vi "VI Tree.vi"   [LabVIEW 2025, in "Chroma 19052.lvlib"]
doc: "This is the instrument driver for the <INSTRUMENT NAME>. The VI Tree displays all the user-callable VIs of the instrument driver in an organized table."
uses:
  <instrlib>/Chroma 19052/Chroma 19052.lvlib
panel:
  # "(c) 2014 <Enter Company Name Here>.  ALL RIGHTS RESERVED."
  # "SEE DIAGRAM\nFOR VI TREE."
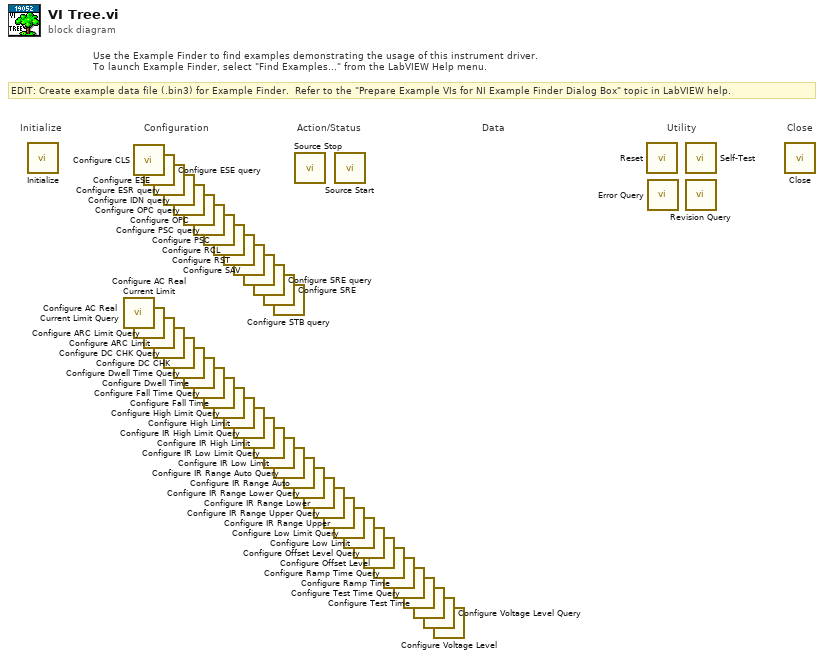
[diagram p0: block diagram]
diagram:
  # "EDIT: Create example data file (.bin3) for Example Finder.  Refer to the \"Prepare Example VIs for NI Example Finder Dialog Box\" topic in LabVIEW help."
  # "Use the Example Finder to find examples demonstrating the usage of this instrument driver.\nTo launch Example Finder, select \"Find Examples...\" from the LabVIEW Help menu."
  # "Configuration"
  # "Utility"
  # "Data"
  # "Action/Status"
  # "Close"
  # "Initialize"
  n1 = call <instrlib>:"Initialize.vi"() -> ()  [unwired: 10 in, 2 out]
  n2 = call <instrlib>:"Configure AC Real Current Limit Query.vi"() -> ()  [unwired: 8 in, 3 out]
  n3 = call <instrlib>:"Configure CLS.vi"() -> ()  [unwired: 10 in, 2 out]
  n4 = call <instrlib>:"Configure AC Real Current Limit.vi"() -> ()  [unwired: 9 in, 2 out]
  n5 = call <instrlib>:"Configure ESE query.vi"() -> ()  [unwired: 9 in, 3 out]
  n6 = call <instrlib>:"Configure ARC Limit Query.vi"() -> ()  [unwired: 9 in, 3 out]
  n7 = call <instrlib>:"Configure ESE.vi"() -> ()  [unwired: 10 in, 2 out]
  n8 = call <instrlib>:"Configure ARC Limit.vi"() -> ()  [unwired: 10 in, 2 out]
  n9 = call <instrlib>:"Configure ESR query.vi"() -> ()  [unwired: 9 in, 3 out]
  n10 = call <instrlib>:"Configure DC CHK Query.vi"() -> ()  [unwired: 10 in, 2 out]
  n11 = call <instrlib>:"Configure IDN query.vi"() -> ()  [unwired: 9 in, 3 out]
  n12 = call <instrlib>:"Configure DC CHK.vi"() -> ()  [unwired: 10 in, 2 out]
  n13 = call <instrlib>:"Configure OPC query.vi"() -> ()  [unwired: 9 in, 3 out]
  n14 = call <instrlib>:"Configure Dwell Time Query.vi"() -> ()  [unwired: 9 in, 3 out]
  n15 = call <instrlib>:"Configure OPC.vi"() -> ()  [unwired: 10 in, 2 out]
  n16 = call <instrlib>:"Configure Dwell Time.vi"() -> ()  [unwired: 10 in, 2 out]
  n17 = call <instrlib>:"Configure PSC query.vi"() -> ()  [unwired: 9 in, 3 out]
  n18 = call <instrlib>:"Configure Fall Time Query.vi"() -> ()  [unwired: 9 in, 3 out]
  n19 = call <instrlib>:"Configure PSC.vi"() -> ()  [unwired: 10 in, 2 out]
  n20 = call <instrlib>:"Configure Fall Time.vi"() -> ()  [unwired: 10 in, 2 out]
  n21 = call <instrlib>:"Configure RCL.vi"() -> ()  [unwired: 10 in, 2 out]
  n22 = call <instrlib>:"Configure High Limit Query.vi"() -> ()  [unwired: 9 in, 3 out]
  n23 = call <instrlib>:"Configure RST.vi"() -> ()  [unwired: 10 in, 2 out]
  n24 = call <instrlib>:"Configure High Limit.vi"() -> ()  [unwired: 10 in, 2 out]
  n25 = call <instrlib>:"Configure SAV.vi"() -> ()  [unwired: 10 in, 2 out]
  n26 = call <instrlib>:"Configure IR High Limit Query.vi"() -> ()  [unwired: 9 in, 3 out]
  n27 = call <instrlib>:"Configure SRE query.vi"() -> ()  [unwired: 9 in, 3 out]
  n28 = call <instrlib>:"Configure IR High Limit.vi"() -> ()  [unwired: 10 in, 2 out]
  n29 = call <instrlib>:"Configure SRE.vi"() -> ()  [unwired: 10 in, 2 out]
  n30 = call <instrlib>:"Configure IR Low Limit Query.vi"() -> ()  [unwired: 9 in, 3 out]
  n31 = call <instrlib>:"Configure STB query.vi"() -> ()  [unwired: 9 in, 3 out]
  n32 = call <instrlib>:"Configure IR Low Limit.vi"() -> ()  [unwired: 10 in, 2 out]
  n33 = call <instrlib>:"Configure IR Range Auto Query.vi"() -> ()  [unwired: 9 in, 3 out]
  n34 = call <instrlib>:"Configure IR Range Auto.vi"() -> ()  [unwired: 10 in, 2 out]
  n35 = call <instrlib>:"Source Stop.vi"() -> ()  [unwired: 10 in, 2 out]
  n36 = call <instrlib>:"Configure IR Range Lower Query.vi"() -> ()  [unwired: 9 in, 3 out]
  n37 = call <instrlib>:"Configure IR Range Lower.vi"() -> ()  [unwired: 10 in, 2 out]
  n38 = call <instrlib>:"Configure IR Range Upper Query.vi"() -> ()  [unwired: 9 in, 3 out]
  n39 = call <instrlib>:"Configure IR Range Upper.vi"() -> ()  [unwired: 10 in, 2 out]
  n40 = call <instrlib>:"Source Start.vi"() -> ()  [unwired: 10 in, 2 out]
  n41 = call <instrlib>:"Configure Low Limit Query.vi"() -> ()  [unwired: 9 in, 3 out]
  n42 = call <instrlib>:"Configure Low Limit.vi"() -> ()  [unwired: 10 in, 2 out]
  n43 = call <instrlib>:"Configure Offset Level Query.vi"() -> ()  [unwired: 10 in, 2 out]
  n44 = call <instrlib>:"Configure Offset Level.vi"() -> ()  [unwired: 10 in, 2 out]
  n45 = call <instrlib>:"Configure Ramp Time Query.vi"() -> ()  [unwired: 9 in, 3 out]
  n46 = call <instrlib>:"Configure Ramp Time.vi"() -> ()  [unwired: 10 in, 2 out]
  n47 = call <instrlib>:"Configure Test Time Query.vi"() -> ()  [unwired: 9 in, 3 out]
  n48 = call <instrlib>:"Configure Test Time.vi"() -> ()  [unwired: 10 in, 2 out]
  n49 = call <instrlib>:"Configure Voltage Level Query.vi"() -> ()  [unwired: 9 in, 3 out]
  n50 = call <instrlib>:"Configure Voltage Level.vi"() -> ()  [unwired: 10 in, 2 out]
  n51 = call <instrlib>:"Reset.vi"() -> ()  [unwired: 10 in, 2 out]
  n52 = call <instrlib>:"Error Query.vi"() -> ()  [unwired: 8 in, 4 out]
  n53 = call <instrlib>:"Self-Test.vi"() -> ()  [unwired: 8 in, 4 out]
  n54 = call <instrlib>:"Revision Query.vi"() -> ()  [unwired: 8 in, 4 out]
  n55 = call <instrlib>:"Close.vi"() -> ()  [unwired: 11 in, 1 out]
